vi "Part-1.vi"() -> ()   [LabVIEW 2015]
panel:
  out "Rectangular":cdb
  in  "Phase":dbl
  in  "Magnitude":dbl
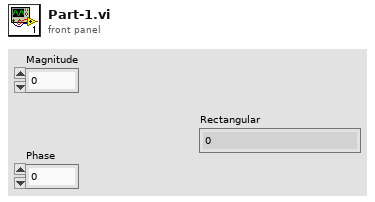
[diagram p1: front panel]
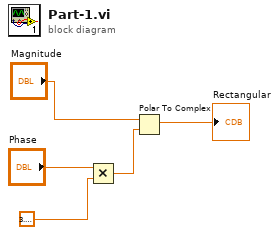
[diagram p0: block diagram]
diagram:
  n1 = Multiply(x="Phase", y=3.141592653589793) -> (x*y=w1:dbl)
  n2 = Polar To Complex(1:w1, 2:"Magnitude") -> (0:→"Rectangular":cdb)
